vi "Plug_in_ADV.vi"() -> (5 "Plug in titles":string[](array[string]), 7 "Plug in values":string[](array[string]))   [LabVIEW 2010]
uses:
  Controls/Post_Process.ctl
  Globals/Meas_global.vi
  Globals/Plug_in_data_global.vi
panel:
  in  "Case Constant\n(See Context Help)":bool=TRUE
  in  "Approx period":dbl format="%.2f"
  in  "End chop":i32
  in  "Start chop":i32
  out "Auto End Chop":i32
  out "Product":dbl[][](graph)
  out "U N0088":dbl[][](graph)
  out "U 1325":dbl[][](graph)
  out "N0088 Auto correlation":T1(graph)
  out "1325 Auto correlation":cluster{dbl, dbl, dbl[]}[](graph)
  out "Correlation Coefficient":T2(graph)
  out "Clipped length":i32
  out "Auto Start Chop":i32
  out "V components":cluster{dbl[], dbl[]}[](graph)
  out "U components":cluster{dbl[], dbl[]}[](graph)
  # "End chop"
  # "End chop"
  # "Amount N0088 lags 1325"
  # "End chop"
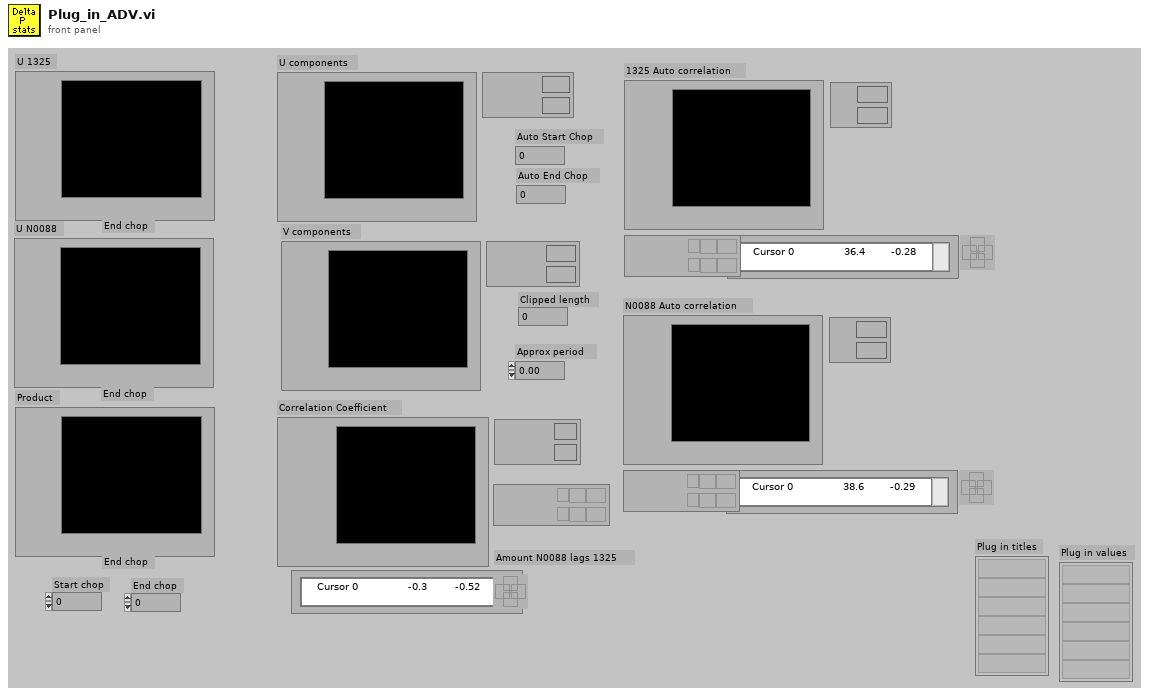
[diagram p1: front panel]
types:
  T1 = cluster{dbl, dbl, "Normalised Auto corr":dbl[]}[]
  T2 = cluster{"Time":dbl[], "Correlation Coefficient":dbl[]}[]
  T3 = typedef "Post_Process.ctl" = enum16{"Take New Data", "Post Process Raw Data File"}
  T4 = typedef "Analysis_info_cluster.ctl" = cluster{"Colour":u32, "Inst type":T5, "Inst name":string, "Symbol":string, "Code name":string, "Extra Info":string, "Inst Array":T6, "Index":i32, "Voltage Index":i32, "Extra Titles":string[], "Extra Values":string[]}
  T5 = typedef "Inst_type.ctl" = enum16{"Propeller anemometer", "Raw voltage", "Pressure Transducer", "Pitot-static tube", "Preston tube", "Hot wire", "Cross wire 1", "Cross wire 2", "Generic Linear", "Generic Polynomial", "Generic BackPoly", "Fast FID", "Thermocouple", "Cold wire", "Pulsed Wire", "LDA Vel", "LDA Tran time", "LDA Arr time"}
  T6 = typedef "Instrument_Array.ctl" = enum16{"PWA", "LDA", "Analogue"}
  T7 = cluster{"Time":dbl[], "Correlation Coefficient":dbl[]}
  T8 = cluster{"Name":string, "X":dbl, "Y":dbl, "Z":dbl}[]
  T9 = cluster{"Name":string, "X":dbl, "Y":dbl, "Z":dbl}
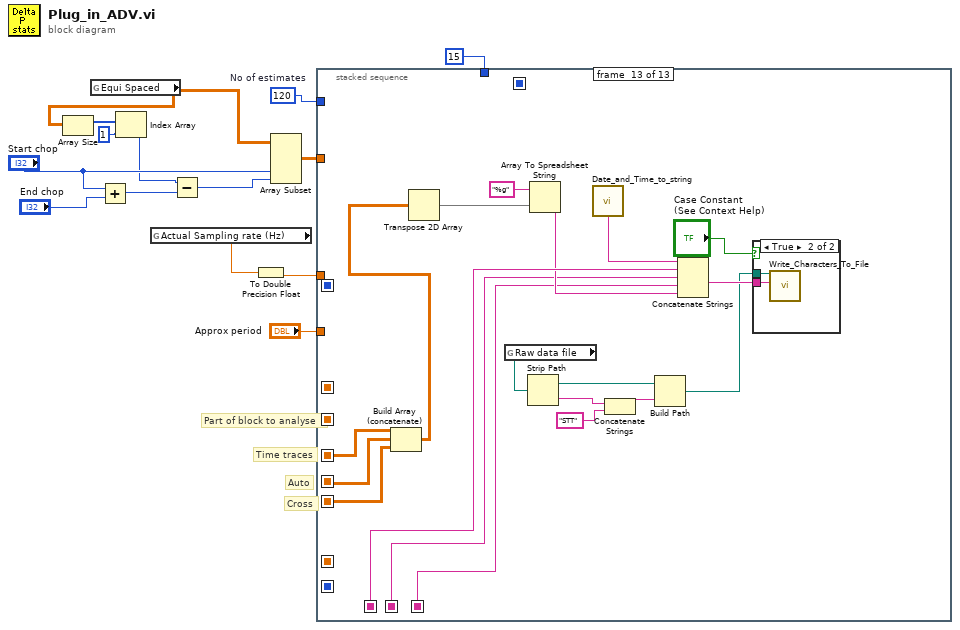
[diagram p0: block diagram]
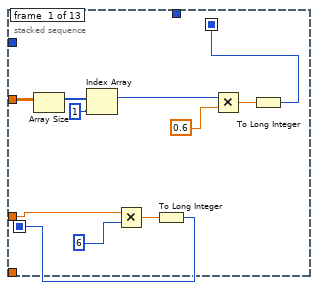
[diagram p2: hidden frame]
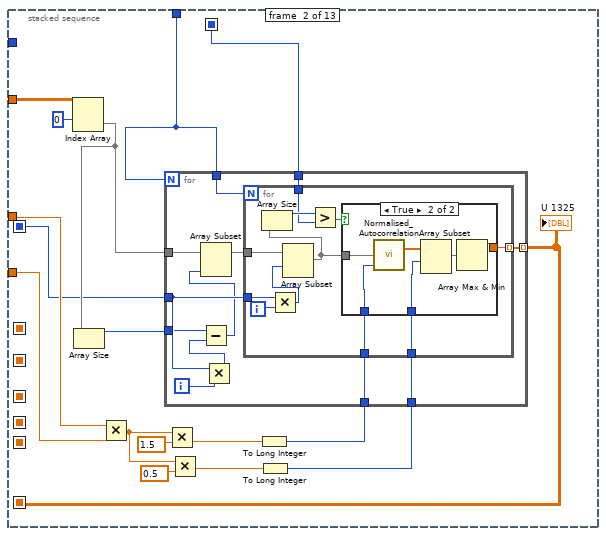
[diagram p3: hidden frame]
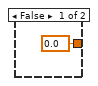
[diagram p4: hidden frame]
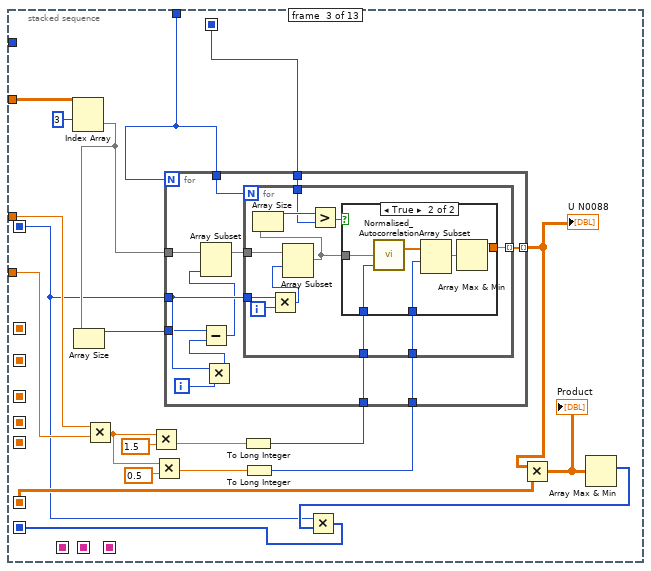
[diagram p5: hidden frame]
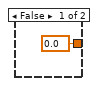
[diagram p6: hidden frame]
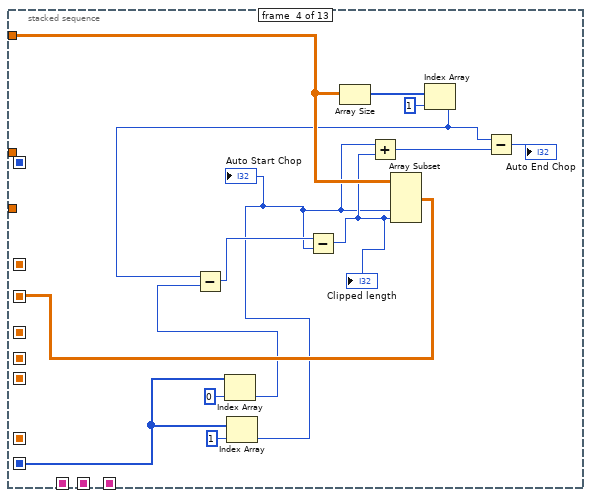
[diagram p7: hidden frame]
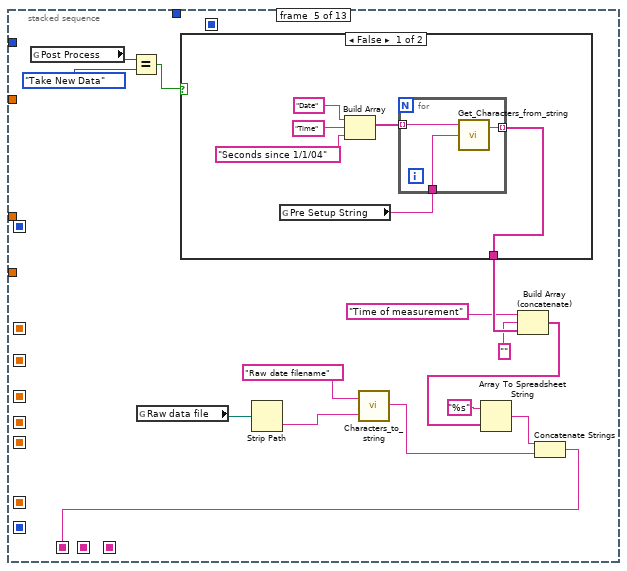
[diagram p8: hidden frame]
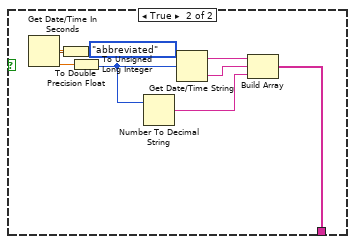
[diagram p9: hidden frame]
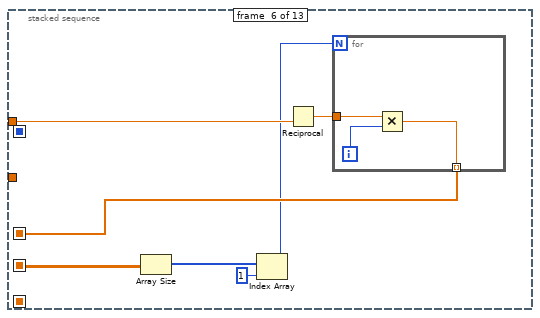
[diagram p10: hidden frame]
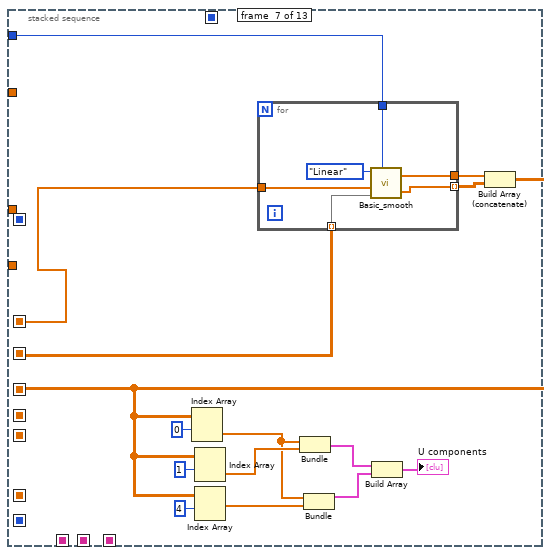
[diagram p11: hidden frame]
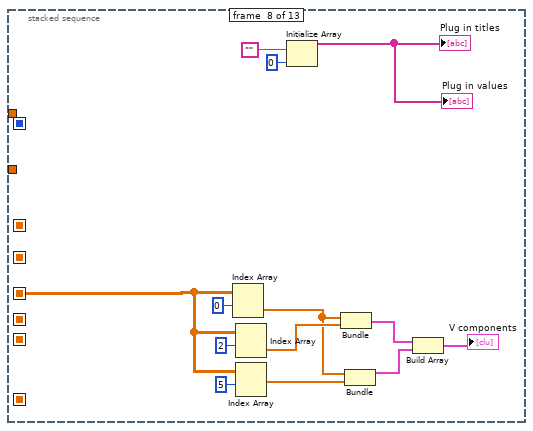
[diagram p12: hidden frame]
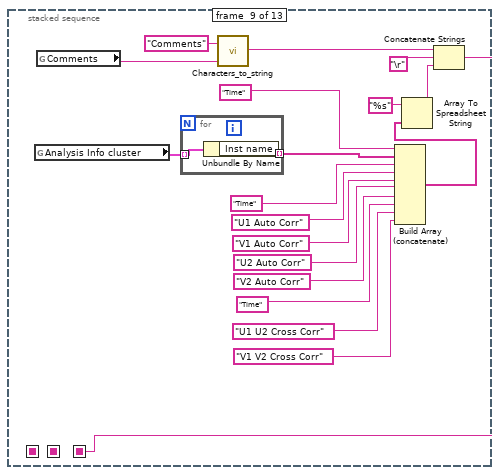
[diagram p13: hidden frame]
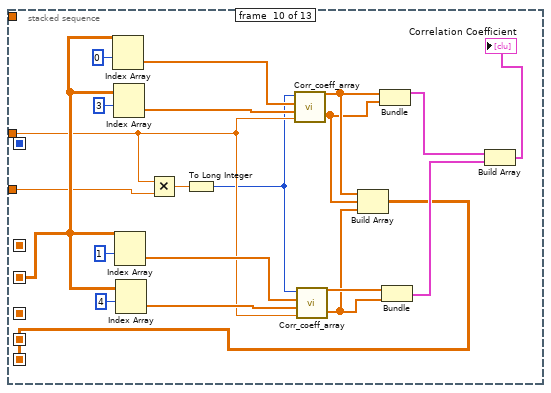
[diagram p14: hidden frame]
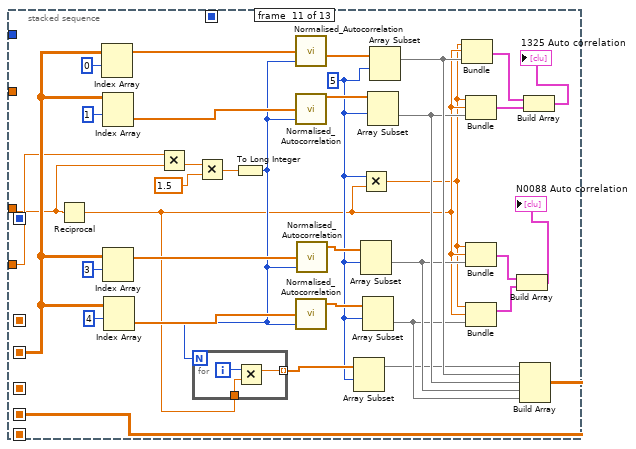
[diagram p15: hidden frame]
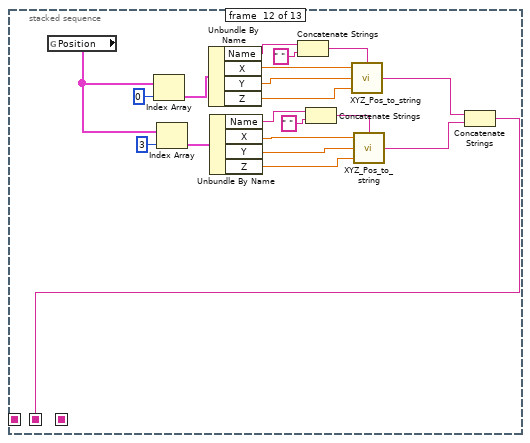
[diagram p16: hidden frame]
diagram:
  w14 = 120  # No of estimates
  # "Cross"
  # "Auto"
  # "Part of block to analyse"
  # "Time traces"
  n1 = global read "Plug_in_data_global.vi" "Equi Spaced"() -> (w8:dbl[][])
  n2 = Array Size(array=w8) -> (size(s)=w9:i32[])
  n3 = Add(x="Start chop", y="End chop") -> (x+y=w4:i32)
  n4 = Index Array(array=w9, index=1) -> (element=w5:i32)
  n5 = global read "Meas_global.vi" "Actual Sampling rate (Hz)"() -> (w13:dbl)
  n6 = Subtract(x=w5, y=w4) -> (x-y=w3:i32)
  n7 = To Double Precision Float(number=w13) -> (double precision float=w12:dbl)
  n8 = Array Subset(array=w8, index (col)="Start chop", length (col)=w3) -> (w11:dbl[][])  [unwired: 2 in]
  n9 = stacked-sequence {
    seq-local: [_ _ _ _ _ _ _ _ w227 _ _ _ _] -> [_ _ _ _ _ _ _ _ _ _ _ _ w320]
    seq-local: [_ _ _ _ _ w174 _ _ _ _ _ _ _] -> [_ _ _ _ _ _ w193 _ _ _ _ _ _]
    seq-local: [_ _ _ _ _ _ w184 _ _ _ _ _ _] -> [_ _ _ _ _ _ _ w201 _ _ _ _ w326]
    seq-local: [_ _ _ _ w144 _ _ _ _ _ _ _ _] -> [_ _ _ _ _ _ _ _ _ _ _ _ w330]
    seq-local: [_ _ _ w137 _ _ _ _ _ _ _ _ _] -> [_ _ _ _ _ w170 w189 _ _ w244 w280 _ _]
    seq-local: [_ _ _ _ _ _ _ _ _ _ w274 _ _] -> [_ _ _ _ _ _ _ _ _ _ _ _ w325]
    seq-local: [_ _ _ _ _ _ _ _ _ w240 _ _ _] -> [_ _ _ _ _ _ _ _ _ _ _ _ w324]
    seq-local: [_ w38 _ _ _ _ _ _ _ _ _ _ _] -> [_ _ w91 _ _ _ _ _ _ _ _ _ _]
    seq-local: [_ _ w88 _ _ _ _ _ _ _ _ _ _] -> [_ _ _ w130 _ _ _ _ _ _ _ _ _]
    seq-local: [_ _ _ _ _ _ _ _ _ _ _ w298 _] -> [_ _ _ _ _ _ _ _ _ _ _ _ w319]
    seq-local: [w16 _ _ _ _ _ _ _ _ _ _ _ _] -> [_ w37 w84 _ _ _ _ _ _ _ _ _ _]
    seq-local: [w15 _ _ _ _ _ _ _ _ _ _ _ _] -> [_ w26 w73 _ _ _ _ _ _ _ _ _ _]
    tunnel: w12 -> [w18 w28 w80 _ _ w173 _ _ _ w236 w272 _ _]
    tunnel: w14 -> [_ _ _ _ _ _ w190 _ _ _ _ _ _]
    tunnel: w11 -> [w19 w41 w92 w136 _ _ _ _ _ _ _ _ _]
    tunnel: "Approx period" -> [_ w29 w81 _ _ _ _ _ _ w237 w273 _ _]
    tunnel: 15 -> [_ w27 w74 _ _ _ _ _ _ _ _ _ _]
    frame #0 {
      n10 = Array Size(array=w19) -> (size(s)=w21:i32[])
      n11 = Index Array(array=w21, index=1) -> (element=w17:i32)
      n12 = Multiply(x=w18, y=6) -> (x*y=w24:dbl)
      n13 = To Long Integer(number=w24) -> (32bit integer=w15:i32)
      n14 = Multiply(x=w17, y=0.6) -> (x*y=w23:dbl)
      n15 = To Long Integer(number=w23) -> (32bit integer=w16:i32)
    }
    frame #1 {
      n16 = Index Array(array=w41, index (row)=0) -> (element=w40:dbl[])  [unwired: 1 in]
      n17 = Array Size(array=w40) -> (size(s)=w39:i32)
      n18 = Multiply(x=w28, y=w29) -> (x*y=w33:dbl)
      n19 = Multiply(x=w33, y=1.5) -> (x*y=w35:dbl)
      n20 = Multiply(x=w33, y=0.5) -> (x*y=w32:dbl)
      n21 = To Long Integer(number=w35) -> (32bit integer=w31:i32)
      n22 = To Long Integer(number=w32) -> (32bit integer=w30:i32)
      n23 = for {
        N: w27 -> [_]
        tunnel: w26 -> [w52]
        tunnel: w40 -> [w48]
        tunnel: w27 -> [w54]
        tunnel: w39 -> [w51]
        tunnel: [w46] -> w38 mode=indexing
        tunnel: w37 -> [w45]
        tunnel: w31 -> [w44]
        tunnel: w30 -> [w43]
        i -> [w53]
        n24 = Multiply(x=w52, y=w53) -> (x*y=w50:i32)
        n25 = Subtract(x=w51, y=w50) -> (x-y=w49:i32)
        n26 = Array Subset(array=w48, length=w49) -> (w47:dbl[])  [unwired: 1 in]
        n27 = for {
          N: w54 -> [_]
          tunnel: w52 -> [w63]
          tunnel: w47 -> [w62]
          tunnel: [w61] -> w46 mode=indexing
          tunnel: w45 -> [w57]
          tunnel: w44 -> [w56]
          tunnel: w43 -> [w55]
          i -> [w65]
          n28 = Multiply(x=w63, y=w65) -> (x*y=w64:i32)
          n29 = Array Subset(array=w62, index=w64) -> (w60:dbl[])  [unwired: 1 in]
          n30 = Array Size(array=w60) -> (size(s)=w58:i32)
          n31 = Greater?(x=w58, y=w57) -> (0:w59:bool)
          n32 = case shown="True" w59 {
            tunnel: [0.0 w72] -> w61
            tunnel: w60 -> [_ w69]
            tunnel: w56 -> [_ w68]
            tunnel: w55 -> [_ w67]
            frame False {
            }
            frame True {
              n33 = call "Normalised_Autocorrelation.vi"("Autocorrelation length"=w68, "Array"=w69) -> ("Normalised Auto corr"=w71:dbl[])  [unwired: 1 in]
              n34 = Array Subset(array=w71, index=w67) -> (w70:dbl[])  [unwired: 1 in]
              n35 = Array Max & Min(array=w70) -> (max value=w72:dbl)  [unwired: 3 out]
            }
          }
        }
      }
      "U 1325" <- w38
    }
    frame #2 {
      n36 = Index Array(array=w92, index (row)=3) -> (element=w87:dbl[])  [unwired: 1 in]
      n37 = Array Size(array=w87) -> (size(s)=w86:i32)
      n38 = Multiply(x=w80, y=w81) -> (x*y=w77:dbl)
      n39 = Multiply(x=w77, y=1.5) -> (x*y=w82:dbl)
      n40 = Multiply(x=w77, y=0.5) -> (x*y=w76:dbl)
      n41 = To Long Integer(number=w82) -> (32bit integer=w79:i32)
      n42 = To Long Integer(number=w76) -> (32bit integer=w75:i32)
      n43 = for {
        N: w74 -> [_]
        tunnel: w73 -> [w103]
        tunnel: w87 -> [w99]
        tunnel: w74 -> [w105]
        tunnel: w86 -> [w102]
        tunnel: [w97] -> w85 mode=indexing
        tunnel: w84 -> [w96]
        tunnel: w79 -> [w95]
        tunnel: w75 -> [w94]
        i -> [w104]
        n44 = Multiply(x=w103, y=w104) -> (x*y=w101:i32)
        n45 = Subtract(x=w102, y=w101) -> (x-y=w100:i32)
        n46 = Array Subset(array=w99, length=w100) -> (w98:dbl[])  [unwired: 1 in]
        n47 = for {
          N: w105 -> [_]
          tunnel: w103 -> [w114]
          tunnel: w98 -> [w113]
          tunnel: [w112] -> w97 mode=indexing
          tunnel: w96 -> [w108]
          tunnel: w95 -> [w107]
          tunnel: w94 -> [w106]
          i -> [w116]
          n48 = Multiply(x=w114, y=w116) -> (x*y=w115:i32)
          n49 = Array Subset(array=w113, index=w115) -> (w111:dbl[])  [unwired: 1 in]
          n50 = Array Size(array=w111) -> (size(s)=w109:i32)
          n51 = Greater?(x=w109, y=w108) -> (0:w110:bool)
          n52 = case shown="True" w110 {
            tunnel: [0.0 w123] -> w112
            tunnel: w111 -> [_ w120]
            tunnel: w107 -> [_ w119]
            tunnel: w106 -> [_ w118]
            frame False {
            }
            frame True {
              n53 = call "Normalised_Autocorrelation.vi"("Autocorrelation length"=w119, "Array"=w120) -> ("Normalised Auto corr"=w122:dbl[])  [unwired: 1 in]
              n54 = Array Subset(array=w122, index=w118) -> (w121:dbl[])  [unwired: 1 in]
              n55 = Array Max & Min(array=w121) -> (max value=w123:dbl)  [unwired: 3 out]
            }
          }
        }
      }
      "U N0088" <- w85
      n56 = Multiply(x=w85, y=w91) -> (x*y=w90:dbl[][])
      "Product" <- w90
      n57 = Array Max & Min(array=w90) -> (max index (indices)=w89:i32[])  [unwired: 3 out]
      n58 = Multiply(x=w73, y=w89) -> (x*y=w88:i32[])
    }
    frame #3 {
      n59 = Index Array(array=w130, index=0) -> (element=w132:i32)
      n60 = Index Array(array=w130, index=1) -> (element=w127:i32)
      "Auto Start Chop" <- w127
      n61 = Array Size(array=w136) -> (size(s)=w134:i32[])
      n62 = Index Array(array=w134, index=1) -> (element=w126:i32)
      n63 = Subtract(x=w126, y=w132) -> (x-y=w129:i32)
      n64 = Subtract(x=w129, y=w127) -> (x-y=w128:i32)
      "Clipped length" <- w128
      n65 = Add(x=w127, y=w128) -> (x+y=w125:i32)
      n66 = Array Subset(array=w136, index (col)=w127, length (col)=w128) -> (w137:dbl[][])  [unwired: 2 in]
      n67 = Subtract(x=w126, y=w125) -> (x-y=→"Auto End Chop":i32)
    }
    frame #4 {
      n68 = global read "Meas_global.vi" "Post Process"() -> (w150:T3)
      n69 = Equal?(x=w150, y=Post_Process."Take New Data" ("Post Process")) -> (x = y?=w149:bool)
      n70 = global read "Meas_global.vi" "Raw data file"() -> (w139:path)
      n71 = case shown="False" w149 {
        tunnel: [w152 w162] -> w143
        frame False {
          n72 = global read "Meas_global.vi" "Pre Setup String"() -> (w153:string)
          n73 = Build Array("Date", "Time", "Seconds since 1/1/04") -> (w154:string[])
          n74 = for {
            tunnel: w154 -> [w160] mode=indexing
            tunnel: w153 -> [w159]
            tunnel: [w158] -> w152 mode=indexing
            n75 = call "Get_Characters_from_string.vi"("Input string"=w159, "Variable name"=w160) -> ("Value"=w158:string)  [unwired: 1 in, 1 out]
          }
        }
        frame True {
          n76 = Get Date/Time In Seconds() -> (seconds since 1Jan1904=w161:timestamp)
          n77 = To Double Precision Float(number=w161) -> (double precision float=w165:dbl)
          n78 = To Unsigned Long Integer(number=w165) -> (unsigned 32bit integer=w164:u32)
          n79 = Number To Decimal String(number=w164) -> (decimal integer string=w163:string)  [unwired: 1 in]
          n80 = Get Date/Time String(date format (0)=enum16{"short", "long", "abbreviated"}."abbreviated", seconds (now)=w164) -> (date string=w167:string, time string=w166:string)  [unwired: 1 in]
          n81 = Build Array(w167, w166, w163) -> (w162:string[])
        }
      }
      n82 = Strip Path(path=w139) -> (name=w138:string)  [unwired: 1 out]
      n83 = call "Characters_to_string.vi"("Characters to write"=w138, "Label for characters"="Raw date filename") -> ("Output string"=w145:string)
      n84 = Build Array (concatenate)("Time of measurement", "" ("Value"), w143) -> (w140:string[])
      n85 = Array To Spreadsheet String(array=w140, 3:"%s" ("format string")) -> (spreadsheet string=w146:string)  [unwired: 1 in]
      n86 = Concatenate Strings(w146, w145) -> (w144:string)
    }
    frame #5 {
      n87 = Array Size(array=w170) -> (size(s)=w171:i32[])
      n88 = Index Array(array=w171, index=1) -> (element=w169:i32)
      n89 = Reciprocal(x=w173) -> (1/x=w175:dbl)
      n90 = for {
        N: w169 -> [_]
        tunnel: w175 -> [w178]
        tunnel: [w176] -> w174 mode=indexing
        i -> [w177]
        n91 = Multiply(x=w178, y=w177) -> (x*y=w176:dbl)
      }
    }
    frame #6 {
      n92 = for {
        tunnel: w193 -> [w198]
        tunnel: w189 -> [w197] mode=indexing
        tunnel: [w196] -> w192
        tunnel: [w195] -> w191 mode=indexing
        tunnel: w190 -> [w194]
        n93 = call "Basic_smooth.vi"("Smoothing"=enum16{"Linear", "Logarithmic"}."Linear", "X array in"=w198, "Y array in"=w197, "No of estimates output"=w194) -> ("X array Out"=w196:dbl[], "Y array Out"=w195:dbl[])  [unwired: 1 in]
      }
      n94 = Build Array (concatenate)(w192, w191) -> (w184:dbl[][])
      n95 = Index Array(array=w184, index (row)=0) -> (element=w183:dbl[])  [unwired: 1 in]
      n96 = Index Array(array=w184, index (row)=1) -> (element=w186:dbl[])  [unwired: 1 in]
      n97 = Index Array(array=w184, index (row)=4) -> (element=w182:dbl[])  [unwired: 1 in]
      n98 = Bundle(w183, w186) -> (w181:cluster{dbl[], dbl[]})  [unwired: 1 in]
      n99 = Bundle(w183, w182) -> (w180:cluster{dbl[], dbl[]})  [unwired: 1 in]
      n100 = Build Array(w181, w180) -> (→"U components":cluster{dbl[], dbl[]}[])
    }
    frame #7 {
      n101 = Index Array(array=w201, index (row)=0) -> (element=w205:dbl[])  [unwired: 1 in]
      n102 = Index Array(array=w201, index (row)=2) -> (element=w207:dbl[])  [unwired: 1 in]
      n103 = Index Array(array=w201, index (row)=5) -> (element=w204:dbl[])  [unwired: 1 in]
      n104 = Initialize Array("", 0) -> (→"Plug in titles" →"Plug in values":string[])
      n105 = Bundle(w205, w207) -> (w203:cluster{dbl[], dbl[]})  [unwired: 1 in]
      n106 = Bundle(w205, w204) -> (w202:cluster{dbl[], dbl[]})  [unwired: 1 in]
      n107 = Build Array(w203, w202) -> (→"V components":cluster{dbl[], dbl[]}[])
    }
    frame #8 {
      n108 = global read "Meas_global.vi" "Analysis Info cluster"() -> (w226:T4[])
      n109 = global read "Meas_global.vi" "Comments"() -> (w231:string)
      n110 = for {
        tunnel: w226 -> [w233] mode=indexing
        tunnel: [w232] -> w213 mode=indexing
        n111 = Unbundle By Name(w233) -> ("Inst name"=w232:string)
      }
      n112 = call "Characters_to_string.vi"("Characters to write"=w231, "Label for characters"="Comments") -> ("Output string"=w229:string)
      n113 = Build Array (concatenate)("Time", w213, "Time", "U1 Auto Corr", "V1 Auto Corr", "U2 Auto Corr", "V2 Auto Corr", "Time", "U1 U2 Cross Corr", "V1 V2 Cross Corr") -> (w218:string[])
      n114 = Array To Spreadsheet String(array=w218, 3:"%s" ("format string")) -> (spreadsheet string=w215:string)  [unwired: 1 in]
      n115 = Concatenate Strings(w229, "\r", w215) -> (w227:string)
    }
    frame #9 {
      n116 = Index Array(array=w244, index (row)=0) -> (element=w248:dbl[])  [unwired: 1 in]
      n117 = Index Array(array=w244, index (row)=3) -> (element=w247:dbl[])  [unwired: 1 in]
      n118 = Index Array(array=w244, index (row)=1) -> (element=w238:dbl[])  [unwired: 1 in]
      n119 = Index Array(array=w244, index (row)=4) -> (element=w252:dbl[])  [unwired: 1 in]
      n120 = Multiply(x=w236, y=w237) -> (x*y=w235:dbl)
      n121 = To Long Integer(number=w235) -> (32bit integer=w234:i32)
      n122 = call "Corr_coeff_array.vi"("Sampling frequency"=w236, "U2"=w247, "U1"=w248, "Slippage range"=w234) -> ("Correlation Coefficient"=w242:dbl[], "Time"=w243:dbl[])
      n123 = call "Corr_coeff_array.vi"("Sampling frequency"=w236, "U2"=w252, "U1"=w238, "Slippage range"=w234) -> ("Correlation Coefficient"=w241:dbl[], "Time"=w251:dbl[])
      n124 = Build Array(w243, w242, w241) -> (w240:dbl[][])
      n125 = Bundle("Time"=w243, "Correlation Coefficient"=w242) -> (w239:T7)  [unwired: 1 in]
      n126 = Bundle("Time"=w251, "Correlation Coefficient"=w241) -> (w250:T7)  [unwired: 1 in]
      n127 = Build Array(w239, w250) -> (→"Correlation Coefficient":T2)
    }
    frame #10 {
      w257 = 5
      n128 = Reciprocal(x=w272) -> (1/x=w256:dbl)
      n129 = Index Array(array=w280, index (row)=0) -> (element=w285:dbl[])  [unwired: 1 in]
      n130 = Index Array(array=w280, index (row)=1) -> (element=w289:dbl[])  [unwired: 1 in]
      n131 = Index Array(array=w280, index (row)=3) -> (element=w284:dbl[])  [unwired: 1 in]
      n132 = Index Array(array=w280, index (row)=4) -> (element=w281:dbl[])  [unwired: 1 in]
      n133 = Multiply(x=w273, y=w272) -> (x*y=w271:dbl)
      n134 = Multiply(x=w271, y=1.5) -> (x*y=w269:dbl)
      n135 = To Long Integer(number=w269) -> (32bit integer=w260:i32)
      n136 = for {
        N: w260 -> [_]
        tunnel: w256 -> [w291]
        tunnel: [w290] -> w259 mode=indexing
        i -> [w292]
        n137 = Multiply(x=w292, y=w291) -> (x*y=w290:dbl)
      }
      n138 = call "Normalised_Autocorrelation.vi"("Autocorrelation length"=w260, "Array"=w285) -> ("Normalised Auto corr"=w268:dbl[])  [unwired: 1 in]
      n139 = call "Normalised_Autocorrelation.vi"("Autocorrelation length"=w260, "Array"=w289) -> ("Normalised Auto corr"=w265:dbl[])  [unwired: 1 in]
      n140 = call "Normalised_Autocorrelation.vi"("Autocorrelation length"=w260, "Array"=w281) -> ("Normalised Auto corr"=w267:dbl[])  [unwired: 1 in]
      n141 = call "Normalised_Autocorrelation.vi"("Autocorrelation length"=w260, "Array"=w284) -> ("Normalised Auto corr"=w266:dbl[])  [unwired: 1 in]
      n142 = Array Subset(array=w259, index=w257) -> (w258:dbl[])  [unwired: 1 in]
      n143 = Multiply(x=w257, y=w256) -> (x*y=w255:dbl)
      n144 = Array Subset(array=w266, index=w257) -> (w262:dbl[])  [unwired: 1 in]
      n145 = Array Subset(array=w267, index=w257) -> (w261:dbl[])  [unwired: 1 in]
      n146 = Array Subset(array=w265, index=w257) -> (w263:dbl[])  [unwired: 1 in]
      n147 = Array Subset(array=w268, index=w257) -> (w264:dbl[])  [unwired: 1 in]
      n148 = Bundle(w255, w256, w264) -> (w279:cluster{dbl, dbl, dbl[]})  [unwired: 1 in]
      n149 = Bundle(w255, w256, w263) -> (w278:cluster{dbl, dbl, dbl[]})  [unwired: 1 in]
      n150 = Bundle(w255, w256, w262) -> (w277:cluster{dbl, dbl, dbl[]})  [unwired: 1 in]
      n151 = Bundle(w255, w256, w261) -> (w276:cluster{dbl, dbl, dbl[]})  [unwired: 1 in]
      n152 = Build Array(w277, w276) -> (→"N0088 Auto correlation":cluster{dbl, dbl, dbl[]}[])
      n153 = Build Array(w258, w264, w263, w262, w261) -> (w274:dbl[][])
      n154 = Build Array(w279, w278) -> (→"1325 Auto correlation":cluster{dbl, dbl, dbl[]}[])
    }
    frame #11 {
      n155 = global read "Meas_global.vi" "Position"() -> (w310:T8)
      n156 = Index Array(array=w310, index=0) -> (element=w309:T9)
      n157 = Index Array(array=w310, index=3) -> (element=w308:T9)
      n158 = Unbundle By Name(w309) -> ("Name"=w295:string, "X"=w306:dbl, "Y"=w305:dbl, "Z"=w304:dbl)
      n159 = Unbundle By Name(w308) -> ("Name"=w293:string, "X"=w303:dbl, "Y"=w302:dbl, "Z"=w301:dbl)
      n160 = Concatenate Strings(w295, " " ("Output string")) -> (w307:string)
      n161 = Concatenate Strings(w293, " " ("Output string")) -> (w297:string)
      n162 = call "XYZ_Pos_to_string.vi"("Position label"=w307, "Z"=w304, "Y"=w305, "X"=w306) -> ("Output string"=w300:string)
      n163 = call "XYZ_Pos_to_string.vi"("Position label"=w297, "Z"=w301, "Y"=w302, "X"=w303) -> ("Output string"=w299:string)
      n164 = Concatenate Strings(w300, w299) -> (w298:string)
    }
    frame #12 {
      n165 = Build Array (concatenate)(w326, w325, w324) -> (w322:dbl[][])
      n166 = Transpose 2D Array(2D array=w322) -> (transposed array=w331:dbl[][])
      n167 = global read "Meas_global.vi" "Raw data file"() -> (w317:path)
      n168 = Strip Path(path=w317) -> (stripped path=w314:path, name=w316:string)
      n169 = Array To Spreadsheet String(array=w331, 3:"%g" ("format string")) -> (spreadsheet string=w321:string)  [unwired: 1 in]
      n170 = call "Date_and_Time_to_string.vi"() -> ("Date and time (spreadsheet)"=w323:string)
      n171 = Concatenate Strings(w316, "STT") -> (w315:string)
      n172 = Build Path(base path=w314, name or relative path=w315) -> (appended path=w313:path)
      n173 = Concatenate Strings(w323, w330, w319, w320, w321) -> (w328:string)
      n174 = case shown="True" "Case Constant\n(See Context Help)" {
        tunnel: w328 -> [_ w333]
        tunnel: w313 -> [_ w332]
        frame False {
        }
        frame True {
          n175 = call "Write_Characters_To_File.vi"("file path (dialog if empty)"=w332, "character string"=w333) -> ()  [unwired: 6 in, 1 out]
        }
      }
    }
  }
